vi "SubVI_StickyButton_Teleop.vi"(1 "Speedy Input":bool, 2 "Number of milliseconds to wait.\n~20ms precision.":i32=12) -> (0 "Sticky Output":bool)   [LabVIEW 2017]
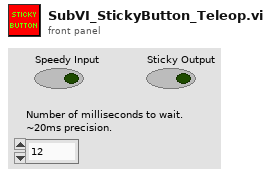
[diagram p1: front panel]
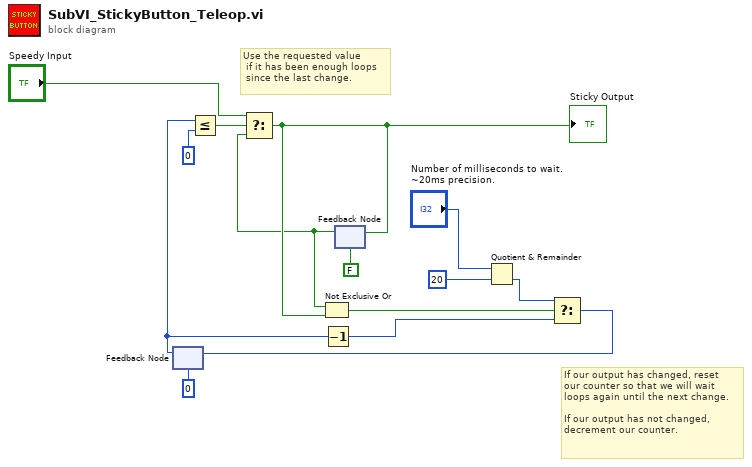
[diagram p0: block diagram]
diagram:
  # "If our output has changed, reset\nour counter so that we will wait \nloops again until the next change.\n\nIf our output has not changed, \ndecrement our counter."
  # "Use the requested value\n if it has been enough loops\n since the last change."
  n1 = feedback #1(0 ("Number of loops to wait \nbetween each change.")) -> (w13:i32)
  n2 = Less Or Equal?(x=w13, y=0 ("x")) -> (x <= y?=w5:bool)
  n3 = Decrement(x=w13) -> (x-1=w8:i32)
  n4 = feedback #2(FALSE ("DriveShifter")) -> (w11:bool)
  n5 = Select(t="Speedy Input", s=w5, f=w11) -> (s? t:f=w14:bool)
  "Sticky Output" <- w14
  n6 = Not Exclusive Or(1:w14, 2:w11) -> (0:w7:bool)
  n7 = feedback-in #2(w14) -> ()
  n8 = Quotient & Remainder(x="Number of milliseconds to wait.\n~20ms precision.", y=20) -> (floor(x/y)=w1:i32)  [unwired: 1 out]
  n9 = Select(t=w1, s=w7, f=w8) -> (s? t:f=w9:i32)
  n10 = feedback-in #1(w9) -> ()
